vi "sub vi - cycle&temp fail v3.vi"(0 "Amps Lo?":bool, 2 "Input Cluster":T1, 3 "SELECT":T2(ring), 4 "Amps Hi?":bool) -> (15 "(FAIL) out":cluster{"FAIL LO":dbl, "FAIL HI":dbl}, 16 "(DISP) out":T3, 17 "(RESULT) out":bool, 19 "file error":errorcluster)   [LabVIEW 2013]
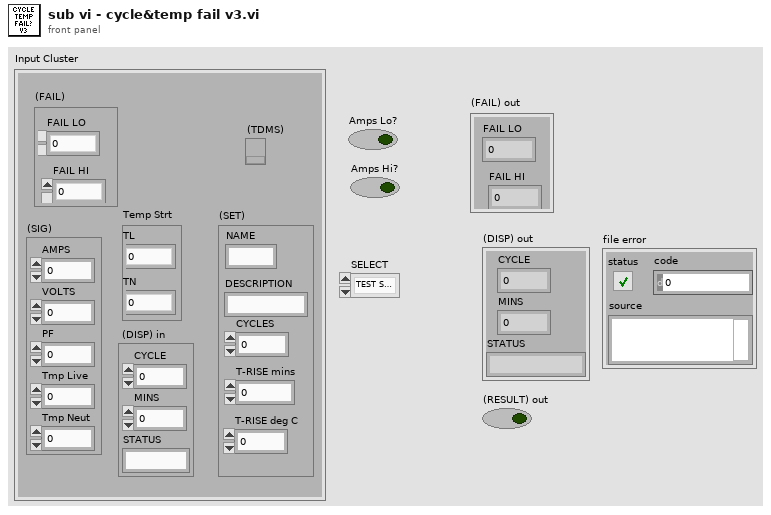
[diagram p1: front panel]
types:
  T1 = cluster{"(FAIL)":cluster{"FAIL LO":dbl, "FAIL HI":dbl}, "(SIG)":cluster{"AMPS":dbl, "VOLTS":dbl, "PF":dbl, "Tmp Live":dbl, "Tmp Neut":dbl}, "Temp Strt":cluster{"TL":dbl, "TN":dbl}, " (DISP) in":cluster{"CYCLE":dbl, "MINS":dbl, "STATUS":string}, "(SET)":cluster{"NAME":string, "DESCRIPTION":string, "CYCLES":dbl, "T-RISE mins":dbl, "T-RISE deg C":dbl}, "(TDMS)":refnum<k34>}
  T2 = enum32{"TEST SET UP", "CYCLE TEST", "T-RISE TEST"}
  T3 = cluster{"CYCLE":dbl, "MINS":dbl, "STATUS":string}
  T4 = cluster{"AMPS":dbl, "VOLTS":dbl, "PF":dbl, "Tmp Live":dbl, "Tmp Neut":dbl}
  T5 = cluster{"NAME":string, "DESCRIPTION":string, "CYCLES":dbl, "T-RISE mins":dbl, "T-RISE deg C":dbl}
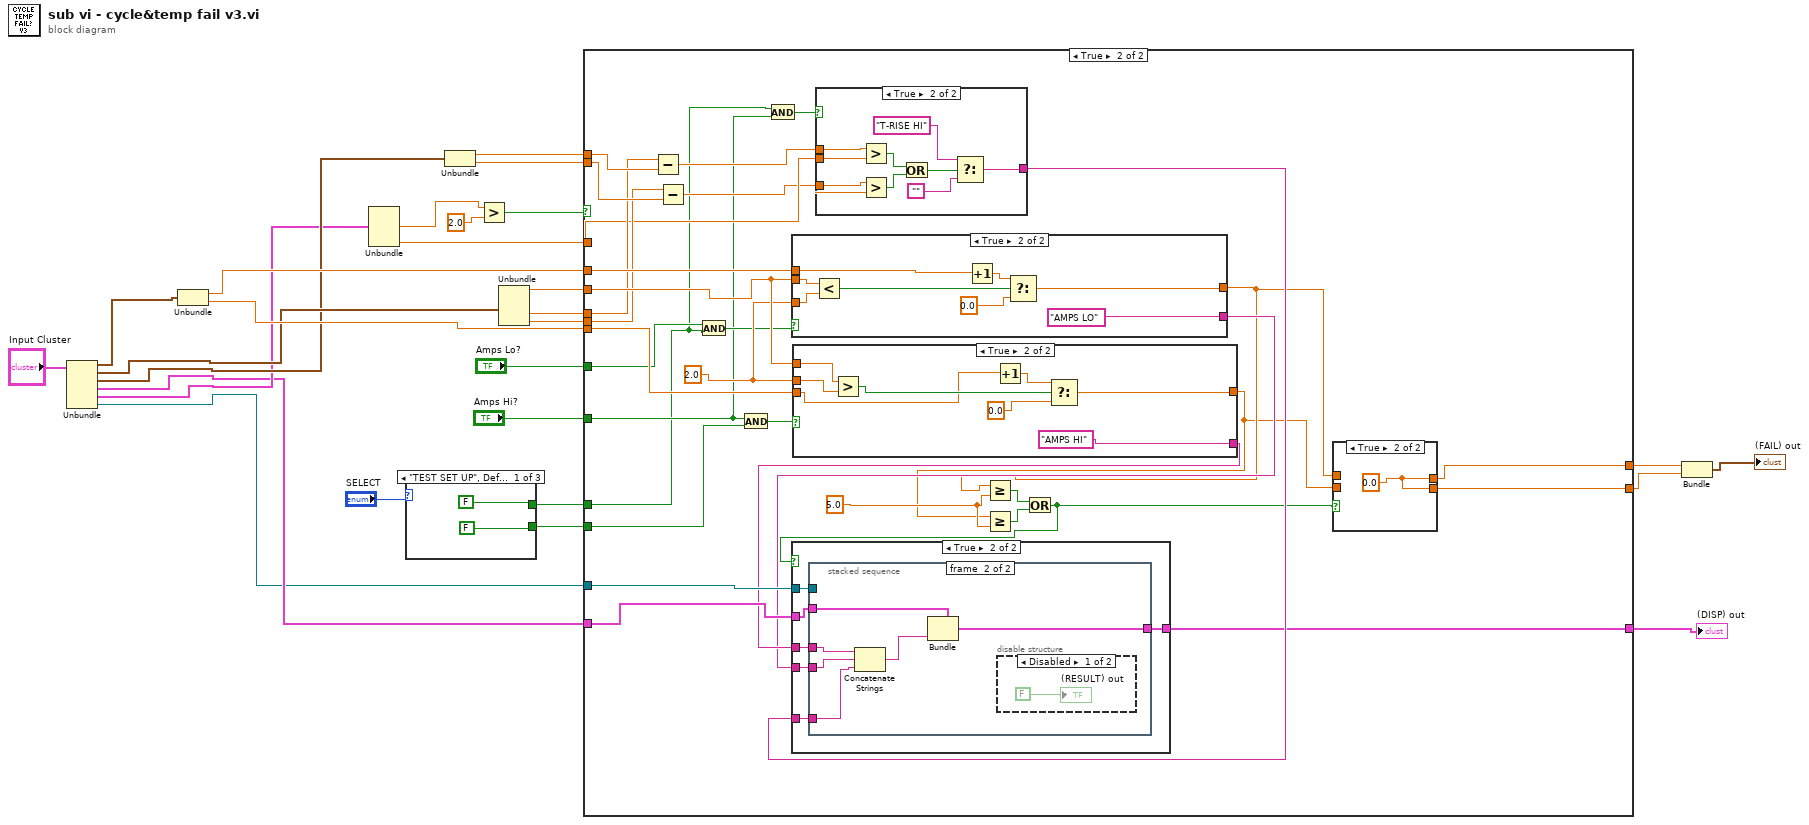
[diagram p0: block diagram]
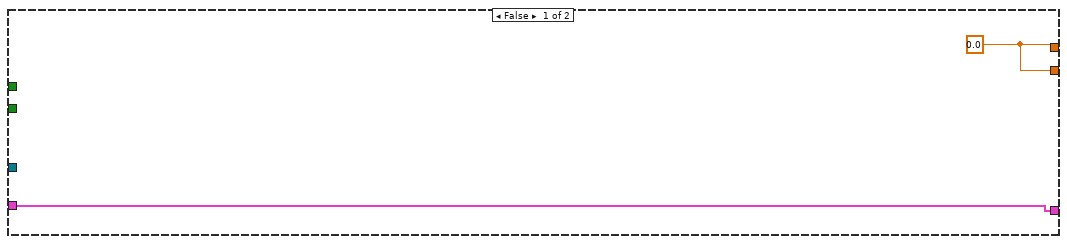
[diagram p2: hidden frame]
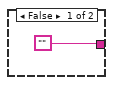
[diagram p4: hidden frame]
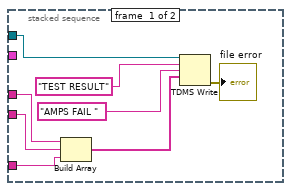
[diagram p6: hidden frame]
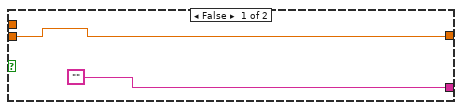
[diagram p8: hidden frame]
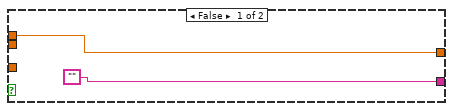
[diagram p9: hidden frame]
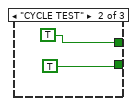
[diagram p10: hidden frame]
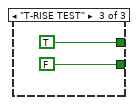
[diagram p11: hidden frame]
diagram:
  n1 = Unbundle("Input Cluster") -> ("(FAIL)"=w12:cluster{"FAIL LO":dbl, "FAIL HI":dbl}, "(SIG)"=w9:T4, "Temp Strt"=w8:cluster{"TL":dbl, "TN":dbl}, "(DISP) in"=w6:T3, "(SET)"=w7:T5, "(TDMS)"=w5:refnum<k34>)
  n2 = Unbundle(w12) -> ("FAIL LO"=w11:dbl, "FAIL HI"=w10:dbl)
  n3 = Unbundle(w7) -> ("CYCLES"=w16:dbl, "T-RISE deg C"=w21:dbl)  [unwired: 3 out]
  n4 = case shown="\"TEST SET UP\", Default" "SELECT" {
    tunnel: [FALSE TRUE TRUE] -> w17
    tunnel: [FALSE TRUE FALSE] -> w20
    frame "TEST SET UP", Default {
    }
    frame "CYCLE TEST" {
    }
    frame "T-RISE TEST" {
    }
  }
  n5 = Unbundle(w8) -> ("TL"=w25:dbl, "TN"=w24:dbl)
  n6 = Greater?(x=w16, y=2.0) -> (0:w14:bool)
  n7 = Unbundle(w9) -> ("AMPS"=w26:dbl, "Tmp Live"=w23:dbl, "Tmp Neut"=w22:dbl)  [unwired: 2 out]
  n8 = case shown="True" w14 {
    tunnel: w26 -> [_ w67]
    tunnel: w11 -> [_ w65]
    tunnel: w10 -> [_ w64]
    tunnel: w5 -> [_ w63]
    tunnel: w6 -> [w34 w62]
    tunnel: w25 -> [_ w61]
    tunnel: w24 -> [_ w60]
    tunnel: w23 -> [_ w59]
    tunnel: w22 -> [_ w58]
    tunnel: w21 -> [_ w57]
    tunnel: w20 -> [_ w47]
    tunnel: "Amps Lo?" -> [_ w45]
    tunnel: "Amps Hi?" -> [_ w43]
    tunnel: w17 -> [_ w42]
    tunnel: [w35 w38] -> w3
    tunnel: [w35 w37] -> w2
    tunnel: [w34 w36] -> w1
    frame False {
      w35 = 0.0
    }
    frame True {
      w50 = 5.0
      w66 = 2.0
      n9 = Subtract(x=w59, y=w61) -> (x-y=w56:dbl)
      n10 = Subtract(x=w58, y=w60) -> (x-y=w55:dbl)
      n11 = And(x=w45, y=w42) -> (x .and. y?=w46:bool)
      n12 = And(x=w43, y=w47) -> (x .and. y?=w48:bool)
      n13 = And(x=w42, y=w43) -> (x .and. y?=w44:bool)
      n14 = case shown="True" w46 {
        tunnel: w67 -> [_ w122]
        tunnel: ["" "AMPS LO"] -> w53
        tunnel: w66 -> [_ w120]
        tunnel: w65 -> [w113 w116]
        tunnel: [w113 w115] -> w41
        frame False {
        }
        frame True {
          n15 = Less?(x=w122, y=w120) -> (x < y?=w119:bool)
          n16 = Increment(x=w116) -> (x+1=w118:dbl)
          n17 = Select(t=w118, s=w119, f=0.0) -> (s? t:f=w115:dbl)
        }
      }
      n18 = case shown="True" w48 {
        tunnel: w67 -> [_ w112]
        tunnel: ["" "AMPS HI"] -> w54
        tunnel: w66 -> [_ w110]
        tunnel: [w103 w106] -> w40
        tunnel: w64 -> [w103 w105]
        frame False {
        }
        frame True {
          n19 = Greater?(x=w112, y=w110) -> (0:w109:bool)
          n20 = Increment(x=w105) -> (x+1=w108:dbl)
          n21 = Select(t=w108, s=w109, f=0.0) -> (s? t:f=w106:dbl)
        }
      }
      n22 = case shown="True" w44 {
        tunnel: w57 -> [_ w80]
        tunnel: w56 -> [_ w79]
        tunnel: w55 -> [_ w78]
        tunnel: ["" w72] -> w49
        frame False {
        }
        frame True {
          n23 = Greater?(x=w79, y=w80) -> (0:w76:bool)
          n24 = Greater?(x=w78, y=w80) -> (0:w77:bool)
          n25 = Or(x=w76, y=w77) -> (x .or. y?=w73:bool)
          n26 = Select(t="T-RISE HI", s=w73, f="") -> (s? t:f=w72:string)
        }
      }
      n27 = Greater Or Equal?(x=w41, y=w50) -> (x >= y?=w52:bool)
      n28 = Greater Or Equal?(x=w40, y=w50) -> (x >= y?=w51:bool)
      n29 = Or(x=w52, y=w51) -> (x .or. y?=w39:bool)
      n30 = case shown="True" w39 {
        tunnel: w54 -> [_ w87]
        tunnel: w53 -> [_ w86]
        tunnel: w62 -> [w81 w85]
        tunnel: w63 -> [_ w84]
        tunnel: w49 -> [_ w83]
        tunnel: [w81 w82] -> w36
        frame False {
        }
        frame True {
          n31 = stacked-sequence {
            tunnel: w87 -> [w94 w101]
            tunnel: w86 -> [w93 w100]
            tunnel: w85 -> [_ w98]
            tunnel: w84 -> [w89 _]
            tunnel: w83 -> [w88 w97]
            tunnel: [_ w96] -> w82
            frame #0 {
              n32 = Build Array(w94, w93, w88) -> (w92:string[])
              n33 = TDMS Write(0:w89, 5:"TEST RESULT", 7:"AMPS FAIL ", 9:w92) -> (15:→"file error":errorcluster)  [unwired: 2 in, 3 out]
            }
            frame #1 {
              n34 = Concatenate Strings(w101, w100, w97) -> (w99:string)
              n35 = Bundle(cluster=w98, "STATUS"=w99) -> (w96:T3)  [unwired: 2 in]
              n36 = disable-structure shown="Disabled" {
                frame Disabled {
                  "(RESULT) out" <- FALSE
                }
                frame Enabled {
                }
              }
            }
          }
        }
      }
      n37 = case shown="True" w39 {
        tunnel: w41 -> [w69 _]
        tunnel: w40 -> [w68 _]
        tunnel: [w69 w70] -> w38
        tunnel: [w68 w70] -> w37
        frame False {
        }
        frame True {
          w70 = 0.0
        }
      }
    }
  }
  "(DISP) out" <- w1
  n38 = Bundle("FAIL LO"=w3, "FAIL HI"=w2) -> (→"(FAIL) out":cluster{"FAIL LO":dbl, "FAIL HI":dbl})  [unwired: 1 in]
